vi "write final cache to tdms.vi"(0 "tdms file in":refnum<k34>, 1 "sample counter":i32, 5 "cache in":T2, 7 "group name":string, 9 "output type order":T3[](array[typedef]), 11 "error in":errorcluster, 12 "scans per write":u16=20, 13 "dictionary":T1) -> (6 "cache out":T2, 15 "error out":errorcluster)   [LabVIEW 2013, in "TDMS datalogger runtime.lvclass"]
uses:
  TDMS datalogger runtime.lvclass
  <vilib>/NI/Tag Bus/tag/Data Type.ctl
  data cache.ctl
  <vilib>/NI/Tag Bus/dictionary/full data dictionary.ctl
  <vilib>/NI/Tag Bus/tag/tag descriptor.lvclass
  <vilib>/NI/Tag Bus/dictionary/data dictionary.lvclass
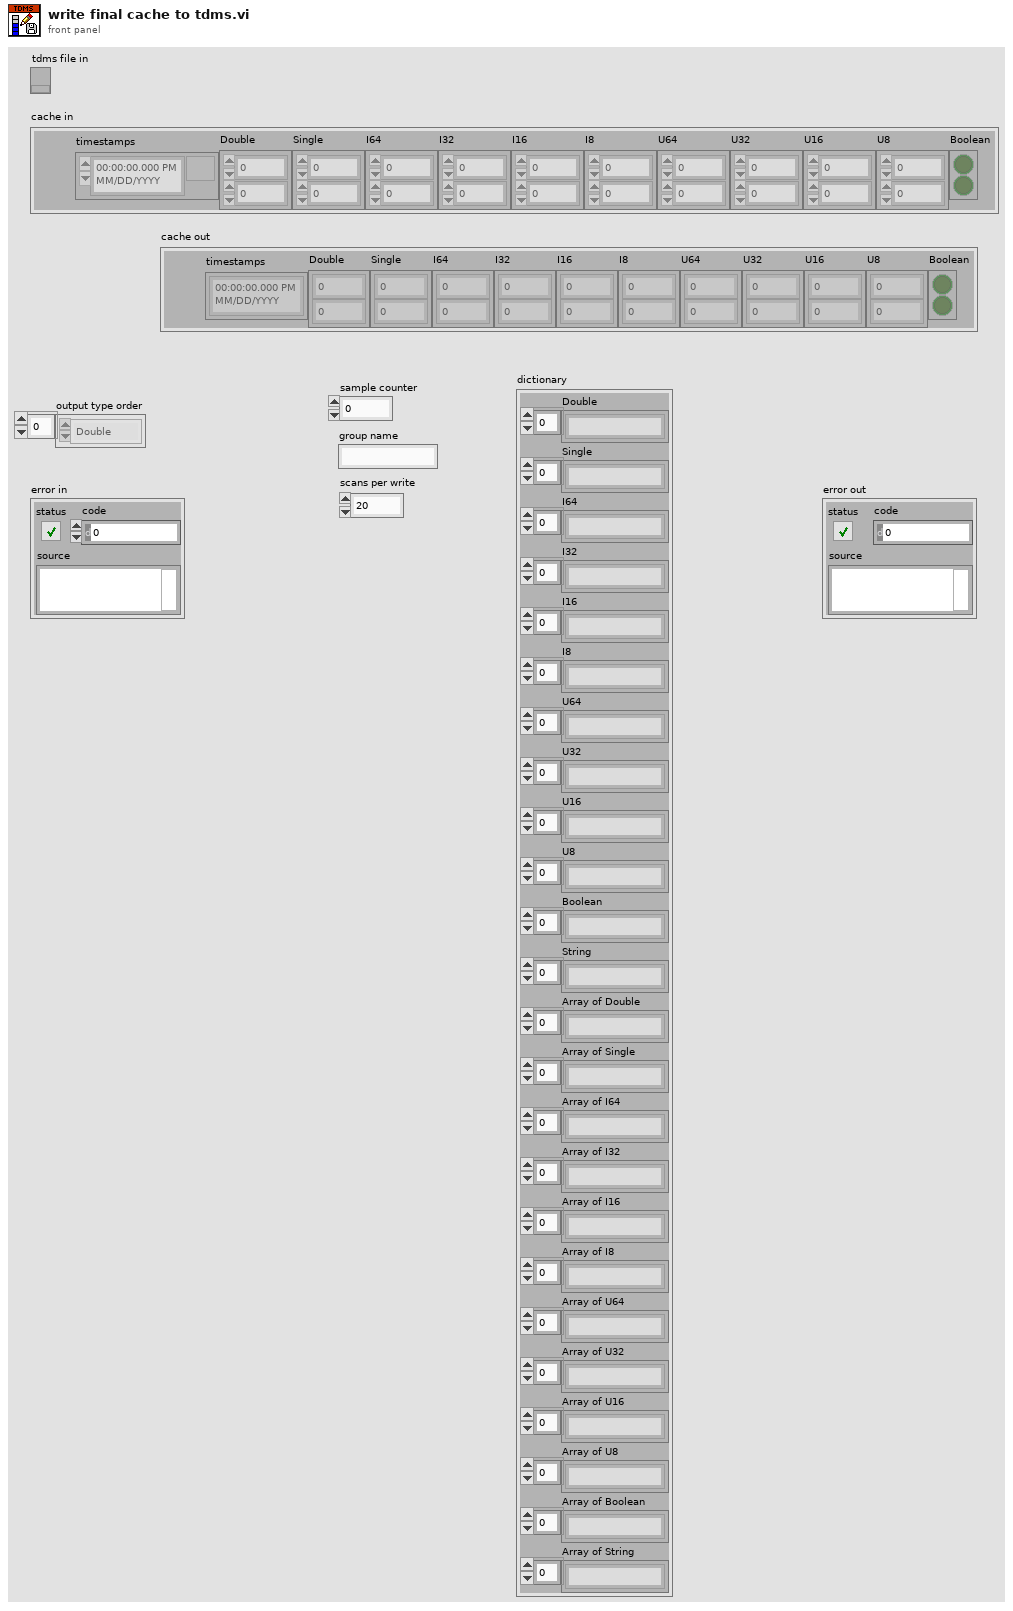
[diagram p1: front panel]
types:
  T1 = typedef "tag bus.lvlib/data dictionary.lvclass/full data dictionary.ctl" = cluster{"Double":string[], "Single":string[], "I64":string[], "I32":string[], "I16":string[], "I8":string[], "U64":string[], "U32":string[], "U16":string[], "U8":string[], "Boolean":string[], "String":string[], "Array of Double":string[], "Array of Single":string[], "Array of I64":string[], "Array of I32":string[], "Array of I16":string[], "Array of I8":string[], "Array of U64":string[], "Array of U32":string[], "Array of U16":string[], "Array of U8":string[], "Array of Boolean":string[], "Array of String":string[]}
  T2 = typedef "TDMS datalogger runtime.lvclass/data cache.ctl" = cluster{"timestamps":timestamp[], "Double":dbl[][], "Single":sgl[][], "I64":i64[][], "I32":i32[][], "I16":i16[][], "I8":i8[][], "U64":u64[][], "U32":u32[][], "U16":u16[][], "U8":u8[][], "Boolean":bool[][]}
  T3 = typedef "tag bus.lvlib/tag descriptor.lvclass/Data Type.ctl" = enum16{"Double", "Single", "I64", "I32", "I16", "I8", "U64", "U32", "U16", "U8", "Boolean", "String", "Array of Double", "Array of Single", "Array of I64", "Array of I32", "Array of I16", "Array of I8", "Array of U64", "Array of U32", "Array of U16", "Array of U8", "Array of Boolean", "Array of String"}
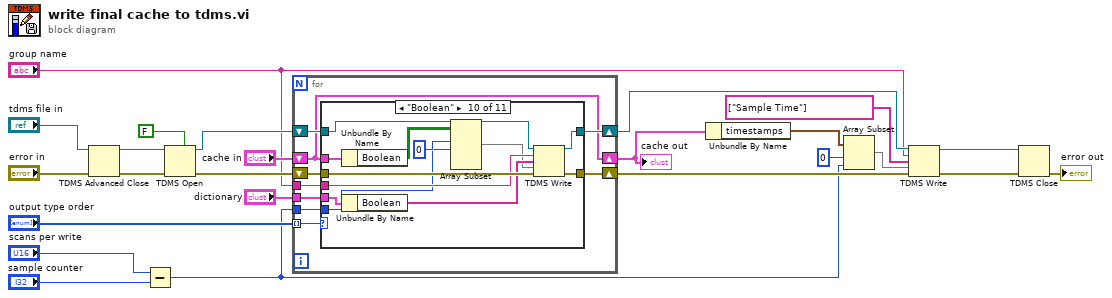
[diagram p0: block diagram]
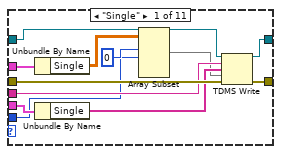
[diagram p2: hidden frame]
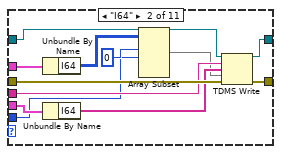
[diagram p3: hidden frame]
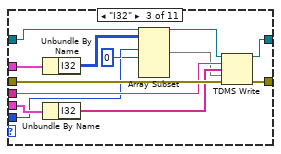
[diagram p4: hidden frame]
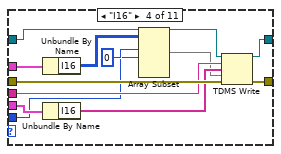
[diagram p5: hidden frame]
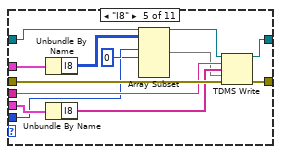
[diagram p6: hidden frame]
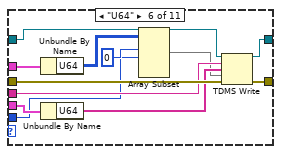
[diagram p7: hidden frame]
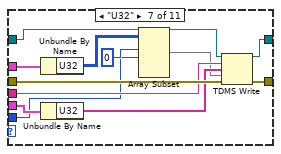
[diagram p8: hidden frame]
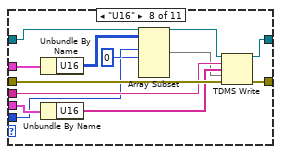
[diagram p9: hidden frame]
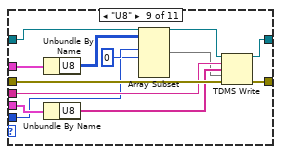
[diagram p10: hidden frame]
diagram:
  n1 = TDMS Advanced Close(8:"error in", 11:"tdms file in") -> (0:w19:errorcluster, 3:w18:path)  [unwired: 2 in]
  n2 = Subtract(x="scans per write", y="sample counter") -> (x-y=w6:i32)
  n3 = TDMS Open(5:FALSE ("create index file? (T)"), 8:w19, 11:w18) -> (0:w15:errorcluster, 3:w16:refnum<k34>)  [unwired: 4 in]
  n4 = for {
    tunnel: "output type order" -> [w30] mode=indexing
    shift-right: [w31] -> w14
    shift-left: w15 -> [w32]
    shift-right: [w29] -> w13
    shift-left: w16 -> [w33]
    shift-right: [w28] -> w22
    shift-left: "cache in" -> [w28]
    tunnel: "dictionary" -> [w27]
    tunnel: "group name" -> [w26]
    tunnel: w6 -> [w25]
    n5 = case shown="\"Boolean\"" w30 {
      tunnel: w33 -> [w40 w52 w64 w76 w88 w100 w112 w124 w136 w148 w154]
      tunnel: w32 -> [w43 w55 w67 w79 w91 w103 w115 w127 w139 w151 w155]
      tunnel: [w42 w54 w66 w78 w90 w102 w114 w126 w138 w150 w155] -> w31
      tunnel: w28 -> [w45 w57 w69 w81 w93 w105 w117 w129 w141 w153 _]
      tunnel: [w41 w53 w65 w77 w89 w101 w113 w125 w137 w149 w154] -> w29
      tunnel: w27 -> [w44 w56 w68 w80 w92 w104 w116 w128 w140 w152 _]
      tunnel: w26 -> [w39 w51 w63 w75 w87 w99 w111 w123 w135 w147 _]
      tunnel: w25 -> [w35 w47 w59 w71 w83 w95 w107 w119 w131 w143 _]
      frame "Single" {
        n6 = Unbundle By Name(w45) -> ("Single"=w37:sgl[][])
        n7 = Unbundle By Name(w44) -> ("Single"=w38:string[])
        n8 = Array Subset(array=w37, index (row)=0 ("index"), length (row)=w35) -> (w34:sgl[][])  [unwired: 2 in]
        n9 = TDMS Write(0:w40, 5:w39, 7:w38, 9:w34, 11:w43) -> (4:w41:refnum<k34>, 15:w42:errorcluster)  [unwired: 1 in, 2 out]
      }
      frame "I64" {
        n10 = Unbundle By Name(w57) -> ("I64"=w49:i64[][])
        n11 = Unbundle By Name(w56) -> ("I64"=w50:string[])
        n12 = Array Subset(array=w49, index (row)=0 ("index"), length (row)=w47) -> (w46:i64[][])  [unwired: 2 in]
        n13 = TDMS Write(0:w52, 5:w51, 7:w50, 9:w46, 11:w55) -> (4:w53:refnum<k34>, 15:w54:errorcluster)  [unwired: 1 in, 2 out]
      }
      frame "I32" {
        n14 = Unbundle By Name(w69) -> ("I32"=w61:i32[][])
        n15 = Unbundle By Name(w68) -> ("I32"=w62:string[])
        n16 = Array Subset(array=w61, index (row)=0 ("index"), length (row)=w59) -> (w58:i32[][])  [unwired: 2 in]
        n17 = TDMS Write(0:w64, 5:w63, 7:w62, 9:w58, 11:w67) -> (4:w65:refnum<k34>, 15:w66:errorcluster)  [unwired: 1 in, 2 out]
      }
      frame "I16" {
        n18 = Unbundle By Name(w81) -> ("I16"=w73:i16[][])
        n19 = Unbundle By Name(w80) -> ("I16"=w74:string[])
        n20 = Array Subset(array=w73, index (row)=0 ("index"), length (row)=w71) -> (w70:i16[][])  [unwired: 2 in]
        n21 = TDMS Write(0:w76, 5:w75, 7:w74, 9:w70, 11:w79) -> (4:w77:refnum<k34>, 15:w78:errorcluster)  [unwired: 1 in, 2 out]
      }
      frame "I8" {
        n22 = Unbundle By Name(w93) -> ("I8"=w85:i8[][])
        n23 = Unbundle By Name(w92) -> ("I8"=w86:string[])
        n24 = Array Subset(array=w85, index (row)=0 ("index"), length (row)=w83) -> (w82:i8[][])  [unwired: 2 in]
        n25 = TDMS Write(0:w88, 5:w87, 7:w86, 9:w82, 11:w91) -> (4:w89:refnum<k34>, 15:w90:errorcluster)  [unwired: 1 in, 2 out]
      }
      frame "U64" {
        n26 = Unbundle By Name(w105) -> ("U64"=w97:u64[][])
        n27 = Unbundle By Name(w104) -> ("U64"=w98:string[])
        n28 = Array Subset(array=w97, index (row)=0 ("index"), length (row)=w95) -> (w94:u64[][])  [unwired: 2 in]
        n29 = TDMS Write(0:w100, 5:w99, 7:w98, 9:w94, 11:w103) -> (4:w101:refnum<k34>, 15:w102:errorcluster)  [unwired: 1 in, 2 out]
      }
      frame "U32" {
        n30 = Unbundle By Name(w117) -> ("U32"=w109:u32[][])
        n31 = Unbundle By Name(w116) -> ("U32"=w110:string[])
        n32 = Array Subset(array=w109, index (row)=0 ("index"), length (row)=w107) -> (w106:u32[][])  [unwired: 2 in]
        n33 = TDMS Write(0:w112, 5:w111, 7:w110, 9:w106, 11:w115) -> (4:w113:refnum<k34>, 15:w114:errorcluster)  [unwired: 1 in, 2 out]
      }
      frame "U16" {
        n34 = Unbundle By Name(w129) -> ("U16"=w121:u16[][])
        n35 = Unbundle By Name(w128) -> ("U16"=w122:string[])
        n36 = Array Subset(array=w121, index (row)=0 ("index"), length (row)=w119) -> (w118:u16[][])  [unwired: 2 in]
        n37 = TDMS Write(0:w124, 5:w123, 7:w122, 9:w118, 11:w127) -> (4:w125:refnum<k34>, 15:w126:errorcluster)  [unwired: 1 in, 2 out]
      }
      frame "U8" {
        n38 = Unbundle By Name(w141) -> ("U8"=w133:u8[][])
        n39 = Unbundle By Name(w140) -> ("U8"=w134:string[])
        n40 = Array Subset(array=w133, index (row)=0 ("index"), length (row)=w131) -> (w130:u8[][])  [unwired: 2 in]
        n41 = TDMS Write(0:w136, 5:w135, 7:w134, 9:w130, 11:w139) -> (4:w137:refnum<k34>, 15:w138:errorcluster)  [unwired: 1 in, 2 out]
      }
      frame "Boolean" {
        n42 = Unbundle By Name(w153) -> ("Boolean"=w145:bool[][])
        n43 = Unbundle By Name(w152) -> ("Boolean"=w146:string[])
        n44 = Array Subset(array=w145, index (row)=0 ("index"), length (row)=w143) -> (w142:bool[][])  [unwired: 2 in]
        n45 = TDMS Write(0:w148, 5:w147, 7:w146, 9:w142, 11:w151) -> (4:w149:refnum<k34>, 15:w150:errorcluster)  [unwired: 1 in, 2 out]
      }
      frame Default {
      }
    }
  }
  "cache out" <- w22
  n46 = Unbundle By Name(w22) -> ("timestamps"=w5:timestamp[])
  n47 = Array Subset(array=w5, index=0, length=w6) -> (w4:timestamp[])
  n48 = TDMS Write(0:w13, 5:"group name", 7:string[] ["Sample Time"] ("channel name(s)"), 9:w4, 11:w14) -> (4:w1:refnum<k34>, 15:w3:errorcluster)  [unwired: 1 in, 2 out]
  n49 = TDMS Close(8:w3, 11:w1) -> (0:→"error out":errorcluster)  [unwired: 1 out]
